vi "host.vi"() -> ()   [LabVIEW 2020]
uses:
  b4957acc-33c7-4f51-b6c8-be02e890b770.vi
  <vilib>/Array/Sort 2D Array - Pop Stack.vi
  <vilib>/Array/Sort 2D Array - Push Stack.vi
  b4957acc-33c7-4f51-b6c8-be02e890b770.vi/269d4b3b-47f5-49e3-8884-44851e4dd9d5.vi
  b4957acc-33c7-4f51-b6c8-be02e890b770.vi/6d99389c-673d-4efb-bf33-19b32bcf4cf8.vi
  <vilib>/FPGAPlugInAG/cRIO-9035/niLvFpga_Open_cRIO-9035.vi
  <vilib>/FPGAPlugInAG/cRIO-9035/niLvFpga_Reset_cRIO-9035.vi
  <vilib>/Utility/error.llb/Error Cluster From Error Code.vi
  <vilib>/rvi/errors/niLvFpgaAdjustHostInterfaceError.vi
  <vilib>/FPGAPlugInAG/cRIO-9035/niLvFpga_Run_cRIO-9035.vi
  <vilib>/FPGAPlugInAG/cRIO-9035/niLvFpga_Close_cRIO-9035.vi
  <vilib>/rvi/interface/nirviOpenFPGA/nirviOpenFPGA.xnode
  FPGA Bitfiles/project_FPGATarget_target_-ZAAaS2nvzc.lvbitx
  target.vi
  <vilib>/rvi/interface/nirviMethod/nirviMethod.xnode
  <vilib>/rvi/interface/nirviReadWriteControl/nirviReadWriteControl.xnode
  <vilib>/rvi/interface/nirviCloseFPGA/nirviCloseFPGA.xnode
  <vilib>/Analysis/NI_AALBase.lvlib
  <vilib>/FPGAPlugInAG/cRIO-9035/niLvFpga_StartFifo_cRIO-9035.vi
  <vilib>/rvi/errors/niLvFpgaMergeErrorWithErrorCode.vi
  <vilib>/FPGAPlugInAG/cRIO-9035/niLvFpga_WriteFifo_cRIO-9035.vi
  <vilib>/FPGAPlugInAG/cRIO-9035/niLvFpga_ReadFifo_cRIO-9035.vi
  NiFpgaLv.dll
panel:
  out "error out":errorcluster
  out "Timed Out? FIFO out index":bool
  out "Timed Out? FIFO out IMG":bool
  out "Timed Out? FIFO out REAL":bool
  out "Timed Out? FIFO in REAL":bool
  out "Timed Out? FIFO in IMG":bool
  out "sorted signal 3":sgl[](graph)
  out "Data":sgl[](array[numeric])
  out "sorted signal 2":sgl[](graph)
  out "index values":i32[](array[numeric])
  out "sorted 2D array":sgl[][](array[numeric])
  out "appended array":sgl[][](array[numeric])
  out "sorted array":sgl[](array[numeric])
  out "uniform white noise":sgl[](array[numeric])
  out "Waveform Graph":sgl[](graph)
  out "sort time (ms)":dbl
  out "Elements Remaining":u32
  out "sorted signal":sgl[](graph)
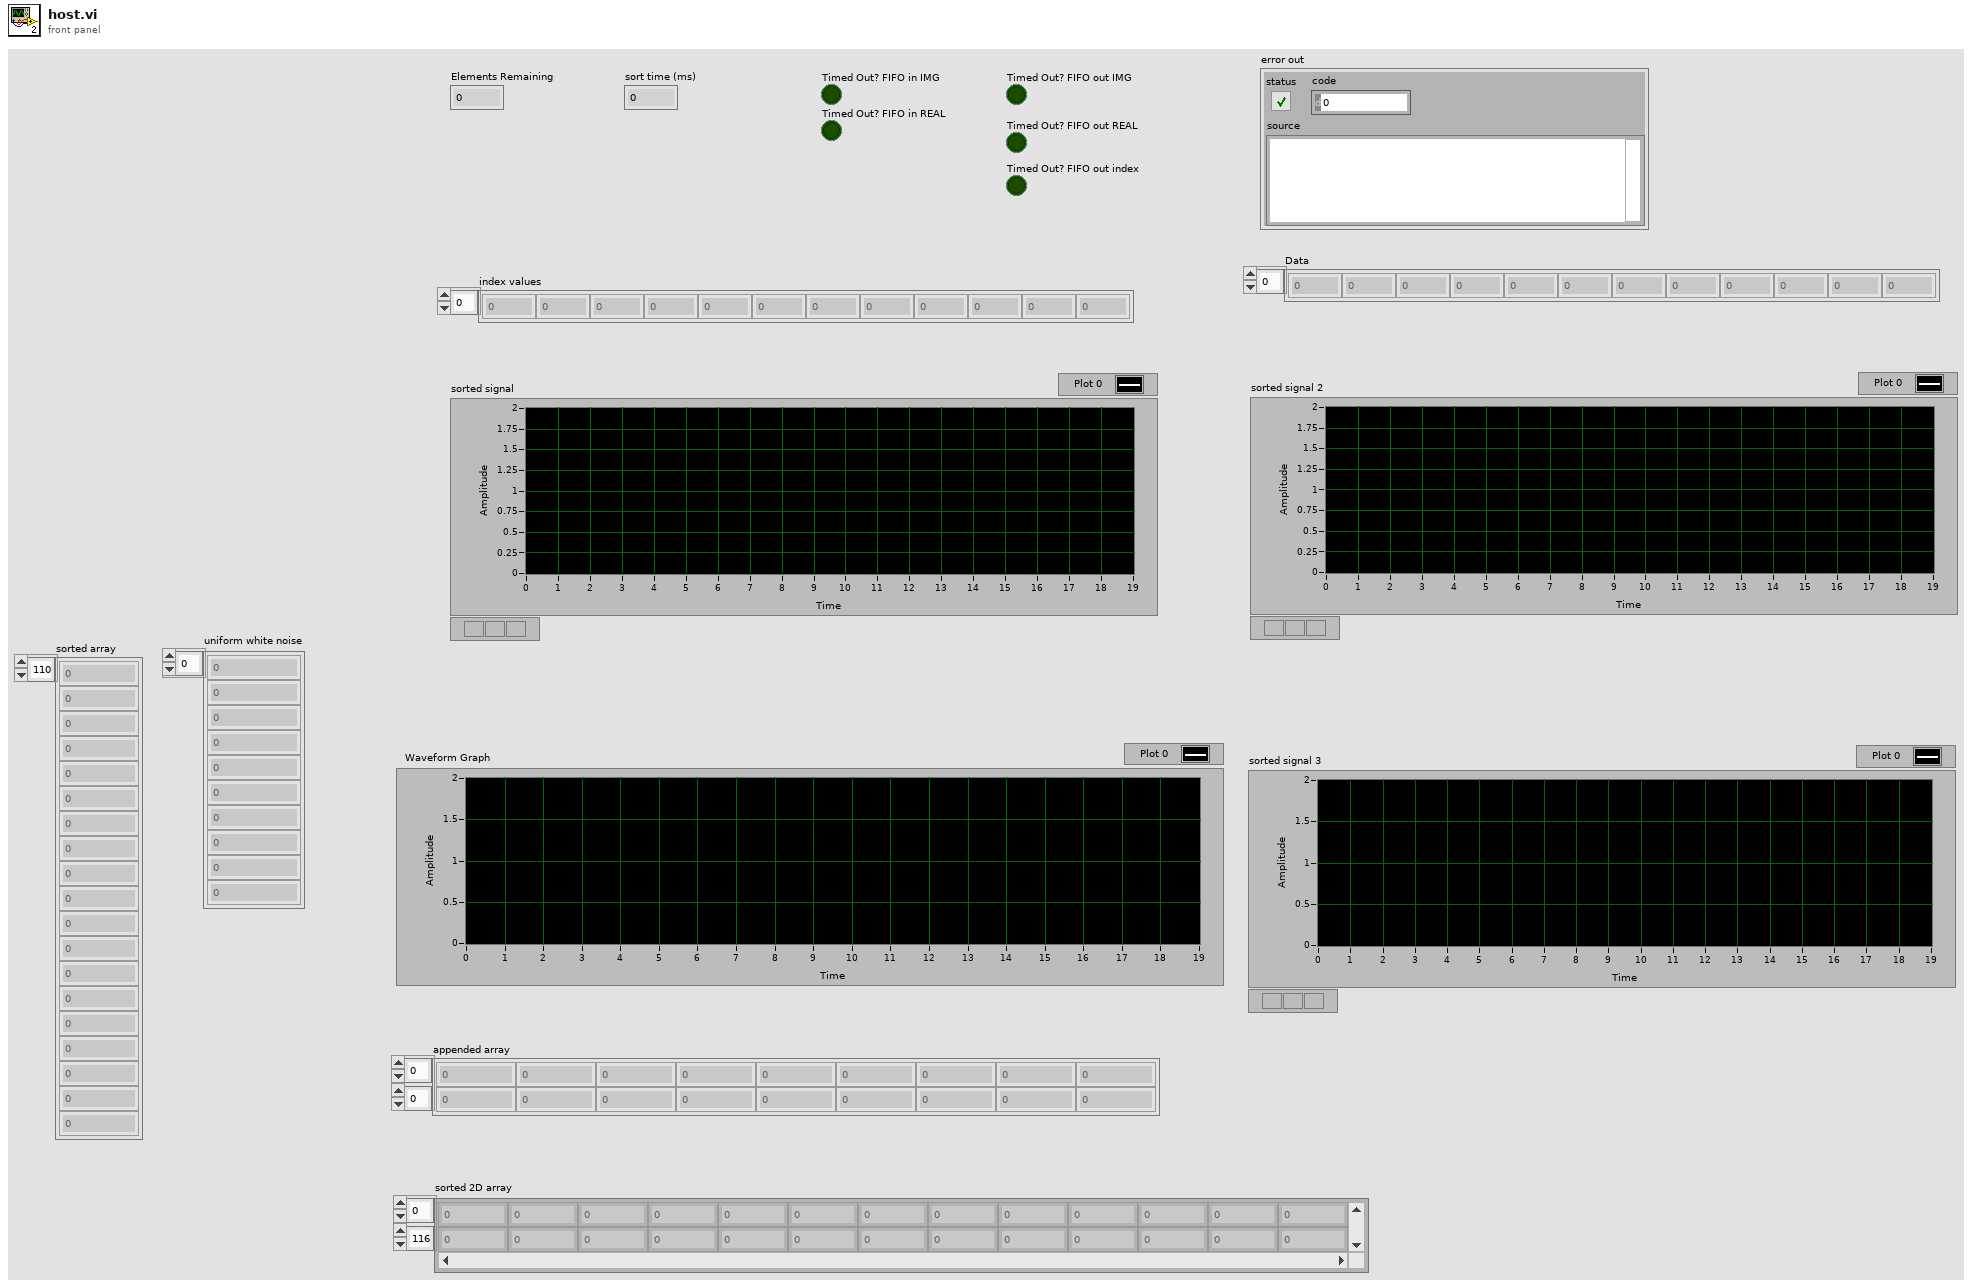
[diagram p1: front panel]
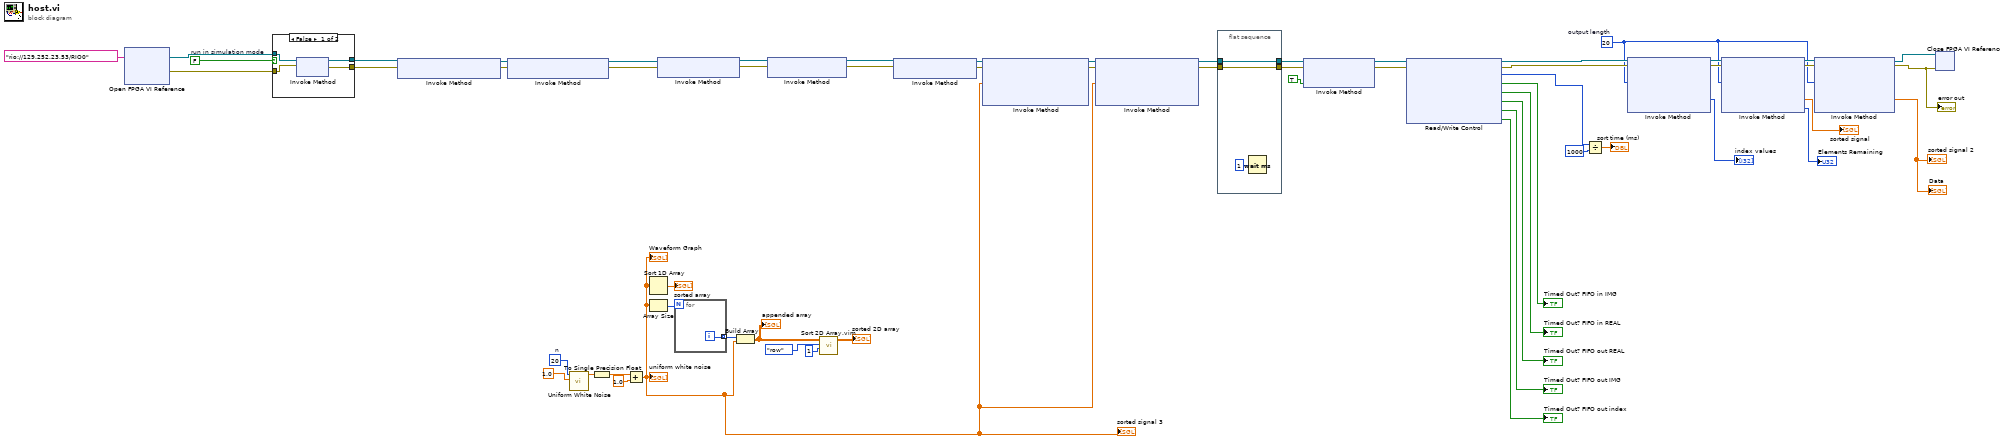
[diagram p0: block diagram]
diagram:
  w6 = FALSE  # run in simulation mode
  w36 = 20  # n
  w23 = u32 20  # output length
  n1 = xnode "Open FPGA VI Reference"("resource name"=tag "rio://129.252.23.53/RIO0") -> ("FPGA VI Reference Out"=w5:refnum<k20>, "error out"=w4:errorcluster)  [unwired: 1 in]
  n2 = case shown="False" w6 {
    tunnel: w5 -> [w63 w64]
    tunnel: w4 -> [w62 w65]
    tunnel: [w61 w64] -> w3
    tunnel: [w60 w65] -> w2
    frame False {
      n3 = xnode "Invoke Method"("FPGA VI Reference In"=w63, "error in"=w62) -> ("FPGA VI Reference Out"=w61:refnum<k20>, "error out"=w60:errorcluster)
    }
    frame True {
    }
  }
  n4 = xnode "Invoke Method"("FPGA VI Reference In"=w3, "error in"=w2) -> ("FPGA VI Reference Out"=w33:refnum<k20>, "error out"=w32:errorcluster)
  n5 = xnode "Invoke Method"("FPGA VI Reference In"=w33, "error in"=w32) -> ("FPGA VI Reference Out"=w18:refnum<k20>, "error out"=w17:errorcluster)
  n6 = call <vilib>:"Uniform White Noise.vi"("amplitude"=1.0, "samples"=w36) -> ("uniform white noise"=w35:dbl[])  [unwired: 8 in, 1 out]
  n7 = To Single Precision Float(number=w35) -> (single precision float=w34:sgl[])
  n8 = Add(x=w34, y=sgl 1.0 ("amplitude")) -> (x+y=w1:sgl[])
  "Waveform Graph" <- w1
  "uniform white noise" <- w1
  "sorted signal 3" <- w1
  n9 = Sort 1D Array(array=w1) -> (sorted array=→"sorted array":sgl[])
  n10 = Array Size(array=w1) -> (size(s)=w42:i32)
  n11 = xnode "Invoke Method"("FPGA VI Reference In"=w18, "error in"=w17) -> ("FPGA VI Reference Out"=w16:refnum<k20>, "error out"=w21:errorcluster)
  n12 = for {
    N: w42 -> [_]
    tunnel: [w66] -> w41 mode=indexing
    i -> [w66]
  }
  n13 = Build Array(w41, w1) -> (w40:sgl[][])
  "appended array" <- w40
  n14 = xnode "Invoke Method"("FPGA VI Reference In"=w16, "error in"=w21) -> ("FPGA VI Reference Out"=w20:refnum<k20>, "error out"=w19:errorcluster)
  n15 = call "Sort 2D Array.vim"("index"=1, "dimension to index (column)"=enum16{"column", "row"}."row", "2D array"=w40) -> ("sorted 2D array"=→"sorted 2D array":sgl[][])  [unwired: 7 in, 1 out]
  n16 = xnode "Invoke Method"("FPGA VI Reference In"=w20, "error in"=w19) -> ("FPGA VI Reference Out"=w31:refnum<k20>, "error out"=w30:errorcluster)
  n17 = xnode "Invoke Method"("FPGA VI Reference In"=w31, "error in"=w30, "Data"=w1) -> ("FPGA VI Reference Out"=w29:refnum<k20>, "error out"=w28:errorcluster)  [unwired: 1 in, 1 out]
  n18 = xnode "Invoke Method"("FPGA VI Reference In"=w29, "error in"=w28, "Data"=w1) -> ("FPGA VI Reference Out"=w9:refnum<k20>, "error out"=w7:errorcluster)  [unwired: 1 in, 1 out]
  n19 = flat-sequence {
    tunnel: [w68] -> w10
    tunnel: w9 -> [w68]
    tunnel: [w67] -> w8
    tunnel: w7 -> [w67]
    frame #0 {
      n20 = Wait (ms)(milliseconds to wait=u32 1) -> ()  [unwired: 1 out]
    }
  }
  n21 = xnode "Invoke Method"("FPGA VI Reference In"=w10, "error in"=w8, "Wait Until Done (F)"=TRUE) -> ("FPGA VI Reference Out"=w56:refnum<k20>, "error out"=w55:errorcluster)
  n22 = xnode "Read/Write Control"("FPGA VI Reference In"=w56, "error in"=w55) -> ("FPGA VI Reference Out"=w50:refnum<k20>, "error out"=w48:errorcluster, "sort time (us)"=w54:u32, "Timed Out? FIFO in IMG"=→"Timed Out? FIFO in IMG":bool, "Timed Out? FIFO in REAL"=→"Timed Out? FIFO in REAL":bool, "Timed Out? FIFO out REAL"=→"Timed Out? FIFO out REAL":bool, "Timed Out? FIFO out IMG"=→"Timed Out? FIFO out IMG":bool, "Timed Out? FIFO out index"=→"Timed Out? FIFO out index":bool)
  n23 = Divide(x=w54, y=u32 1000) -> (x/y=→"sort time (ms)":dbl)
  n24 = xnode "Invoke Method"("FPGA VI Reference In"=w50, "error in"=w48, "Number of Elements"=w23) -> ("FPGA VI Reference Out"=w49:refnum<k20>, "error out"=w47:errorcluster, "Data"=→"index values":i32[])  [unwired: 1 in, 1 out]
  n25 = xnode "Invoke Method"("FPGA VI Reference In"=w49, "error in"=w47, "Number of Elements"=w23) -> ("FPGA VI Reference Out"=w27:refnum<k20>, "error out"=w26:errorcluster, "Data"=→"sorted signal":sgl[], "Elements Remaining"=→"Elements Remaining":u32)  [unwired: 1 in]
  n26 = xnode "Invoke Method"("FPGA VI Reference In"=w27, "error in"=w26, "Number of Elements"=w23) -> ("FPGA VI Reference Out"=w25:refnum<k20>, "error out"=w24:errorcluster, "Data"=→"sorted signal 2" →"Data":sgl[])  [unwired: 1 in, 1 out]
  "error out" <- w24
  n27 = xnode "Close FPGA VI Reference"("FPGA VI Reference In"=w25, "error in"=w24) -> ()  [unwired: 1 out]
